vi "SQLProcedures.vi"(4 "error in (no error)":errorcluster, 6 "ProcName":string, 7 "InputHandle":i32) -> (0 "error out":errorcluster, 3 "OutputHandle":i32)   [LabVIEW 2011]
doc: "Charge la liste des requêtes (fonction du catalogue)"
uses:
  Odbc32.dll
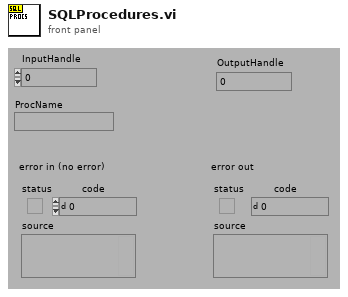
[diagram p1: front panel]
types:
  T1 = enum16{"NOPE", "SQL_HANDLE_ENV", "SQL_HANDLE_DBC", "SQL_HANDLE_STMT", "SQL_HANDLE_DESC"}
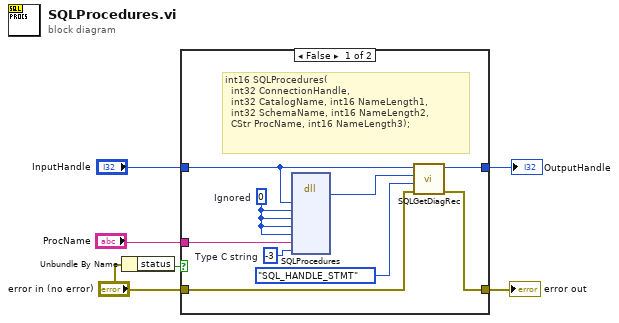
[diagram p0: block diagram]
diagram:
  n1 = Unbundle By Name("error in (no error)") -> ("status"=w2:bool)
  n2 = case shown="False" w2 {
    tunnel: "ProcName" -> [w13 _]
    tunnel: "InputHandle" -> [w12 w17]
    tunnel: [w11 w17] -> w4
    tunnel: [w8 w16] -> w1
    tunnel: "error in (no error)" -> [w9 w16]
    frame False {
      w14 = i16 -3  # Type C string
      w15 = 0  # Ignored
      # "int16 SQLProcedures(\n  int32 ConnectionHandle, \n  int32 CatalogName, int16 NameLength1, \n  int32 SchemaName, int16 NameLength2, \n  CStr ProcName, int16 NameLength3);"
      n3 = dll-call lib="Odbc32.dll" fn="SQLProcedures"("ConnectionHandle"=w12, "CatalogName"=w15, "NameLength1"=w15, "SchemaName"=w15, "NameLength2"=w15, "ProcName"=w13, "NameLength3"=w14) -> (w10:i16)  [unwired: 8 in, 4 out]
      n4 = call "SQLGetDiagRec.vi"("error in (no error)"=w9, "HandleType"=T1."SQL_HANDLE_STMT", "Status (SQL_SUCCESS=0)"=w10, "Input Handle"=w12) -> ("error out"=w8:errorcluster, "Output Handle"=w11:i32)  [unwired: 2 out]
    }
    frame True {
    }
  }
  "OutputHandle" <- w4
  "error out" <- w1
